vi "TLS Client and Server with Self-Signed Server Certificate.vi"() -> ()   [LabVIEW 2023]
doc: "This example demonstrates the use of Start TLS and Accept TLS to secure a TCP connection. A self-signed server certificate is included in the example."
panel:
  out "server error out":errorcluster
  out "client error out":errorcluster
  in  "expected server hostname (must be \"lvtls.example\")":string="lvtls.example"
  in  "Use TLS?":bool=TRUE
  in  "server port":u16=4625
  in  "data sent by server":string="foo"
  out "sent data matches received data?":bool
  out "data received by client":string
  # "Overview: Demonstrates a TLS client and server communicating with each other.\nInstructions:\n1. Set \"Use TLS?\" to FALSE. Run the VI. Communication occurs over unencrypted TCP.\n2. Set \"Use TLS?\" to TRUE. Run the VI. Communication occurs over TLS. The server uses a private key and certificate located next to this VI.\n3. Change the value of \"expected server hostname\". Run the VI. TLS negotiation will fail because the hostname in the server certificate does not match."
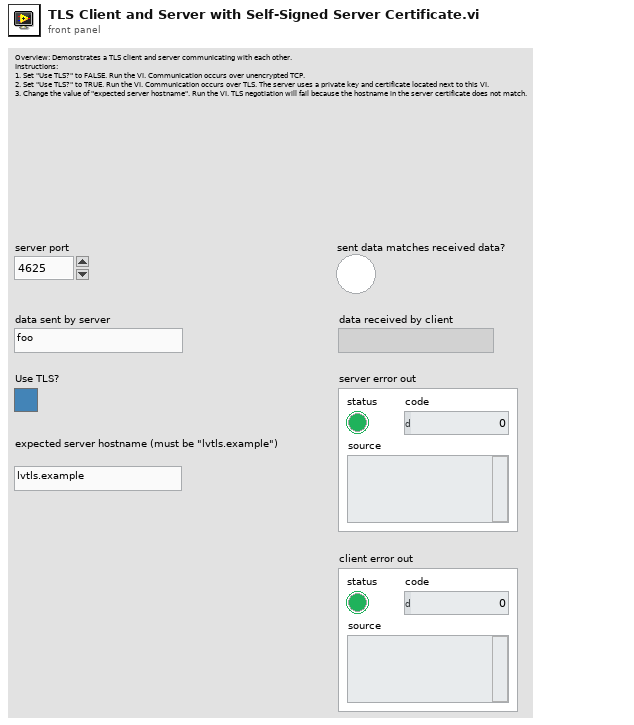
[diagram p1: front panel]
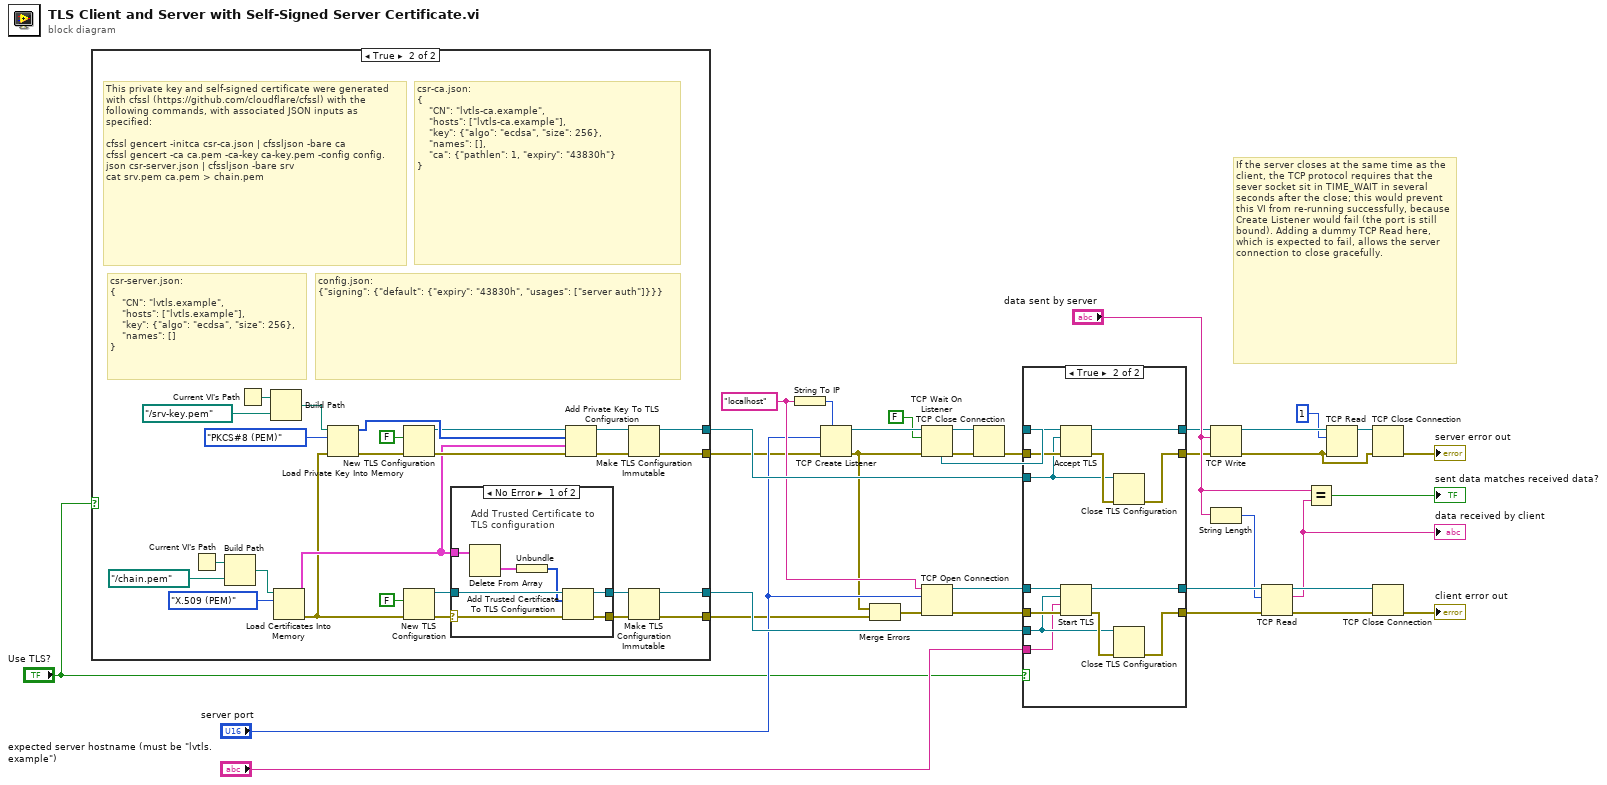
[diagram p0: block diagram]
diagram:
  w23 = "localhost" ("name")
  # "If the server closes at the same time as the client, the TCP protocol requires that the sever socket sit in TIME_WAIT in several seconds after the close; this would prevent this VI from re-running successfully, because Create Listener would fail (the port is still bound). Adding a dummy TCP Read here, which is expected to fail, allows the server connection to close gracefully."
  n1 = case shown="True" "Use TLS?" {
    tunnel: [_ w61] -> w35
    tunnel: [_ w60] -> w24
    tunnel: [_ w59] -> w20
    tunnel: [_ w58] -> w15
    frame False {
    }
    frame True {
      # "config.json:\n{\"signing\": {\"default\": {\"expiry\": \"43830h\", \"usages\": [\"server auth\"]}}}"
      # "csr-server.json:\n{\n    \"CN\": \"lvtls.example\",\n    \"hosts\": [\"lvtls.example\"],\n    \"key\": {\"algo\": \"ecdsa\", \"size\": 256},\n    \"names\": []\n}"
      # "csr-ca.json:\n{\n    \"CN\": \"lvtls-ca.example\",\n    \"hosts\": [\"lvtls-ca.example\"],\n    \"key\": {\"algo\": \"ecdsa\", \"size\": 256},\n    \"names\": [],\n    \"ca\": {\"pathlen\": 1, \"expiry\": \"43830h\"}\n}"
      # "This private key and self-signed certificate were generated with cfssl (https://github.com/cloudflare/cfssl) with the following commands, with associated JSON inputs as specified:\n\ncfssl gencert -initca csr-ca.json | cfssljson -bare ca\ncfssl gencert -ca ca.pem -ca-key ca-key.pem -config config.json csr-server.json | cfssljson -bare srv\ncat srv.pem ca.pem > chain.pem"
      n2 = Current VI's Path() -> (path=w42:path)
      n3 = Build Path(base path=w42, name or relative path=path "../chain.pem" ("cert chain")) -> (appended path=w38:path)
      n4 = Current VI's Path() -> (path=w43:path)
      n5 = Build Path(base path=w43, name or relative path=path "../srv-key.pem" ("key")) -> (appended path=w40:path)
      n6 = Load Certificates Into Memory(10:enum32{"X.509 (PEM)"}."X.509 (PEM)" ("format"), 11:w38) -> (0:w44:errorcluster, 3:w45:cluster{"certificate":u8[]}[])  [unwired: 1 in]
      n7 = Load Private Key Into Memory(8:w44, 10:enum32{"PKCS#8 (PEM)", "PKCS#8 (DER)"}."PKCS#8 (PEM)" ("format"), 11:w40) -> (0:w54:errorcluster, 3:w55:u8[])  [unwired: 1 in]
      n8 = New TLS Configuration(8:w54, 10:FALSE ("load OS trusted CAs?")) -> (0:w52:errorcluster, 3:w53:refnum<k36>)
      n9 = New TLS Configuration(8:w44, 10:FALSE ("load OS trusted CAs?")) -> (0:w46:errorcluster, 3:w47:refnum<k36>)
      n10 = case shown="No Error" w46 {
        selector: w46 -> [w65 w70]
        tunnel: w45 -> [w68 _]
        tunnel: w47 -> [w66 w69]
        tunnel: [w64 w70] -> w48
        tunnel: [w63 w69] -> w49
        frame No Error {
          # "Add Trusted Certificate to\nTLS configuration"
          n11 = Delete From Array(array=w68) -> (deleted portion=w67:cluster{"certificate":u8[]})  [unwired: 2 in, 1 out]
          n12 = Unbundle(w67) -> ("certificate"=w62:u8[])
          n13 = Add Trusted Certificate To TLS Configuration(8:w65, 10:w62, 11:w66) -> (0:w64:errorcluster, 3:w63:refnum<k36>)
        }
        frame Error {
        }
      }
      n14 = Add Private Key To TLS Configuration(8:w52, 9:w45, 10:w55, 11:w53) -> (0:w57:errorcluster, 3:w56:refnum<k36>)
      n15 = Make TLS Configuration Immutable(8:w57, 11:w56) -> (0:w59:errorcluster, 3:w60:refnum<k36>)
      n16 = Make TLS Configuration Immutable(8:w48, 11:w49) -> (0:w58:errorcluster, 3:w61:refnum<k36>)
    }
  }
  n17 = String To IP(1:w23) -> (0:w21:u32)
  n18 = TCP Create Listener(7:w21, 8:w20, 10:"server port") -> (0:w16:errorcluster, 3:w19:refnum<k5>)  [unwired: 2 in, 1 out]
  n19 = Merge Errors(w16, w15) -> (w14:errorcluster)
  n20 = TCP Wait On Listener(8:w16, 10:FALSE ("resolve remote address (T)"), 11:w19) -> (0:w7:errorcluster, 3:w6:refnum<k5>, 4:w17:refnum<k5>)  [unwired: 1 in, 2 out]
  n21 = TCP Open Connection(address=w23, remote port or service name="server port", error in (no error)=w14) -> (connection ID=w33:refnum<k5>, error out=w32:errorcluster)  [unwired: 2 in]
  n22 = TCP Close Connection(connection ID=w6, error in (no error)=w7) -> (error out=w5:errorcluster)  [unwired: 1 in, 1 out]
  n23 = case shown="True" "Use TLS?" {
    tunnel: w35 -> [_ w76]
    tunnel: [w72 w77] -> w34
    tunnel: w33 -> [w72 w87]
    tunnel: w32 -> [w71 w86]
    tunnel: [w74 w85] -> w25
    tunnel: w24 -> [_ w80]
    tunnel: w17 -> [w74 w84]
    tunnel: w5 -> [w73 w83]
    tunnel: [w71 w78] -> w9
    tunnel: [w73 w81] -> w8
    tunnel: "expected server hostname (must be \"lvtls.example\")" -> [_ w75]
    frame False {
    }
    frame True {
      n24 = Accept TLS(8:w83, 10:w80, 11:w84) -> (0:w82:errorcluster, 3:w85:refnum<k5>)  [unwired: 1 in, 1 out]
      n25 = Start TLS(8:w86, 9:w75, 10:w76, 11:w87) -> (0:w79:errorcluster, 3:w77:refnum<k5>)  [unwired: 2 in, 1 out]
      n26 = Close TLS Configuration(8:w82, 11:w80) -> (0:w81:errorcluster)
      n27 = Close TLS Configuration(8:w79, 11:w76) -> (0:w78:errorcluster)
    }
  }
  n28 = TCP Write(connection ID=w25, data in="data sent by server", error in (no error)=w8) -> (connection ID out=w13:refnum<k5>, error out=w10:errorcluster)  [unwired: 1 in, 1 out]
  n29 = String Length(string="data sent by server") -> (length=w26:i32)
  n30 = TCP Read(connection ID=w34, bytes to read=w26, error in (no error)=w9) -> (connection ID out=w31:refnum<k5>, data out=w29:string, error out=w30:errorcluster)  [unwired: 2 in]
  "data received by client" <- w29
  n31 = Equal?(x="data sent by server", y=w29) -> (x = y?=→"sent data matches received data?":bool)
  n32 = TCP Read(connection ID=w13, bytes to read=1, error in (no error)=w10) -> (connection ID out=w12:refnum<k5>)  [unwired: 2 in, 2 out]
  n33 = TCP Close Connection(connection ID=w12, error in (no error)=w10) -> (error out=→"server error out":errorcluster)  [unwired: 1 in, 1 out]
  n34 = TCP Close Connection(connection ID=w31, error in (no error)=w30) -> (error out=→"client error out":errorcluster)  [unwired: 1 in, 1 out]
